vi "Tokenize string on commas.vi"(11 "Unity TCP data received":string) -> (3 "Tokenized Unity Message":string[](array[string]))   [LabVIEW 2024]
panel:
  in  "Empty String Array":string[](array[string])
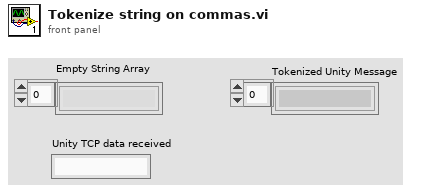
[diagram p1: front panel]
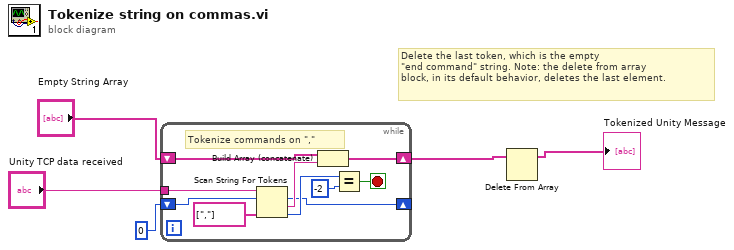
[diagram p0: block diagram]
diagram:
  # "Delete the last token, which is the empty \n\"end command\" string. Note: the delete from array \nblock, in its default behavior, deletes the last element."
  n1 = while {
    tunnel: "Unity TCP data received" -> [w15]
    shift-right: [w10] -> w2
    shift-left: "Empty String Array" -> [w9]
    shift-right: [w6] -> _
    shift-left: 0 ("offset past token") -> [w7]
    stop <- w12 stop-if-true
    # "Tokenize commands on \",\""
    n2 = Scan String For Tokens(6:string[] [","] ("delimiters (\\s,\\t,\\r,\\n)"), 8:w7, 9:w15) -> (0:w8:i32, 1:w11:string, 2:w6:i32)  [unwired: 3 in, 1 out]
    n3 = Build Array (concatenate)(w9, w11) -> (w10:string[])
    n4 = Equal?(x=w8, y=-2) -> (x = y?=w12:bool)
  }
  n5 = Delete From Array(array=w2) -> (array with subset deleted=→"Tokenized Unity Message":string[])  [unwired: 2 in, 1 out]
